vi "PKG_IMC_MoveDist.vi"(4 "axis":i32, 5 "wait":i32, 6 "tgvel":dbl, 7 "endvel":dbl, 9 "startvel":dbl, 10 "dist":i32, 11 "handle":u32) -> (2 "function return":i32, 3 "handle out":u32)   [LabVIEW 2011, in "IMC_Pkg4xxx.lvlib"]
doc: "PKG_IMC_MoveDist(IMC_HANDLE handle, long dist, double startvel, double endvel, double tgvel, int wait, int axis);"
uses:
  IMC_Pkg4xxx.lvlib
  IMC_Pkg4xxx.dll
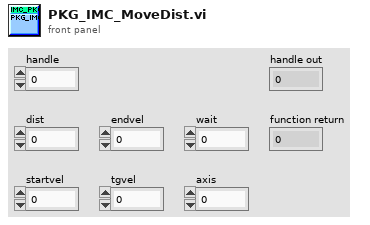
[diagram p1: front panel]
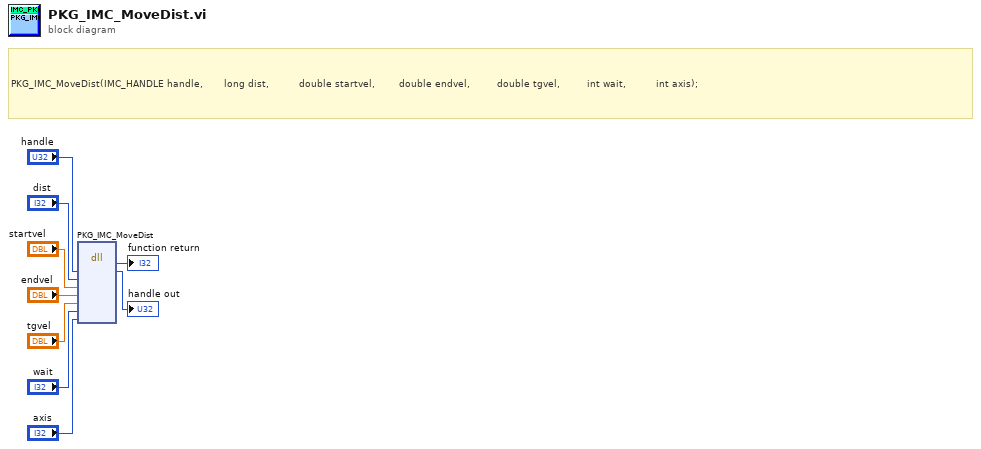
[diagram p0: block diagram]
diagram:
  # "PKG_IMC_MoveDist(IMC_HANDLE handle, \t\t\t\t\t\tlong dist, \t\t\t\t\t\t\t\t\tdouble startvel, \t\t\t\t\t\t\tdouble endvel, \t\t\t\t\t\t\t\tdouble tgvel, \t\t\t\t\t\t\t\tint wait, \t\t\t\t\t\t\t\t\tint axis);"
  n1 = dll-call lib="PTH1mabs F光盘刻录\niMC MotionIMCNet_V4.0IMCAppincLabviewIMC_PKG4xxxIMC_PKG4xxx\nIMC_Pkg4xxx.*" fn="PKG_IMC_MoveDist"("handle"="handle", "dist"="dist", "startvel"="startvel", "endvel"="endvel", "tgvel"="tgvel", "wait"="wait", "axis"="axis") -> (→"function return":i32, "handle"=→"handle out":u32)  [unwired: 9 in, 2 out]
